vi "CalcInbetween.vi"(4 "PointY":dbl(slide) scale=-10.0..10.0, 6 "PointX":dbl(slide) scale=-10.0..10.0, 8 "Line2Y":dbl=4.0, 9 "Line2X":dbl=2.0, 10 "Line1Y":dbl format="%#_13g", 11 "Line1X":dbl format="%#_13g") -> (1 "Inbetween?":bool)   [LabVIEW 2014]
panel:
  out "Angle":dbl
  in  "cluster":T1
  out "XY Graph":cluster{dbl[], dbl[]}[](graph)
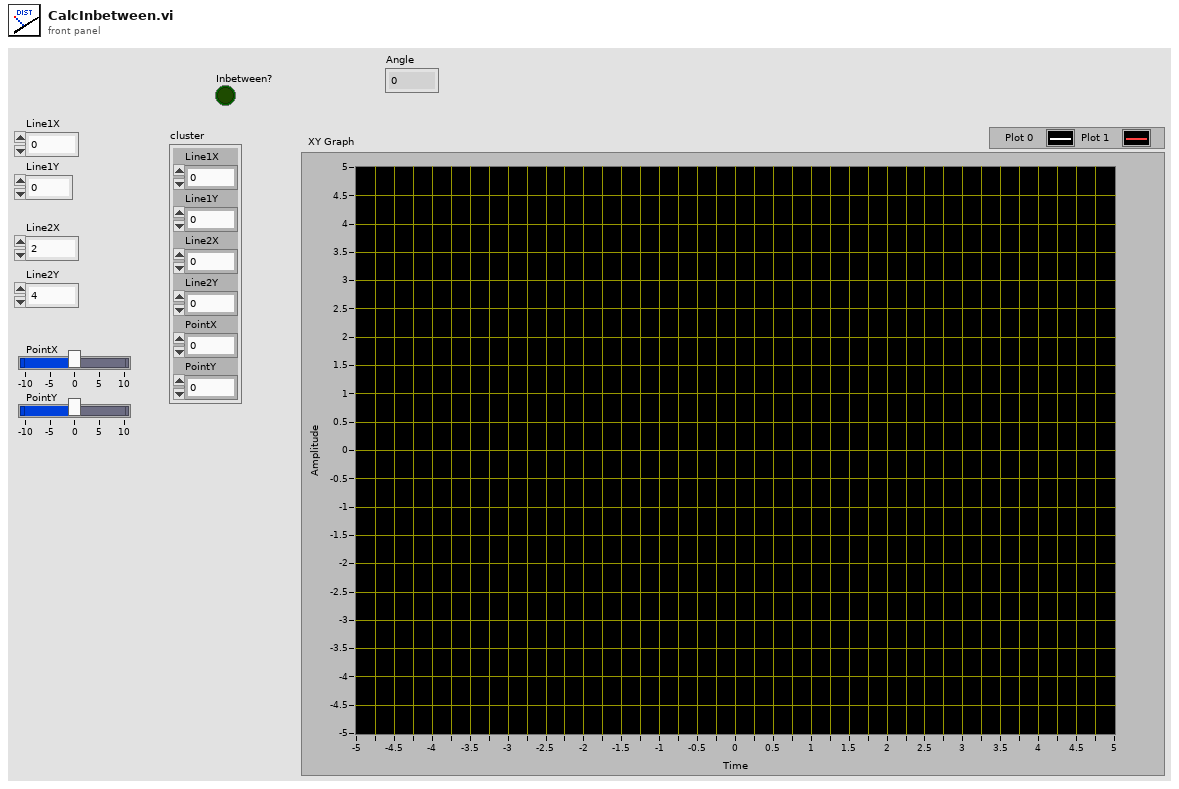
[diagram p1: front panel]
types:
  T1 = cluster{"Line1X":dbl, "Line1Y":dbl, "Line2X":dbl, "Line2Y":dbl, "PointX":dbl, "PointY":dbl}
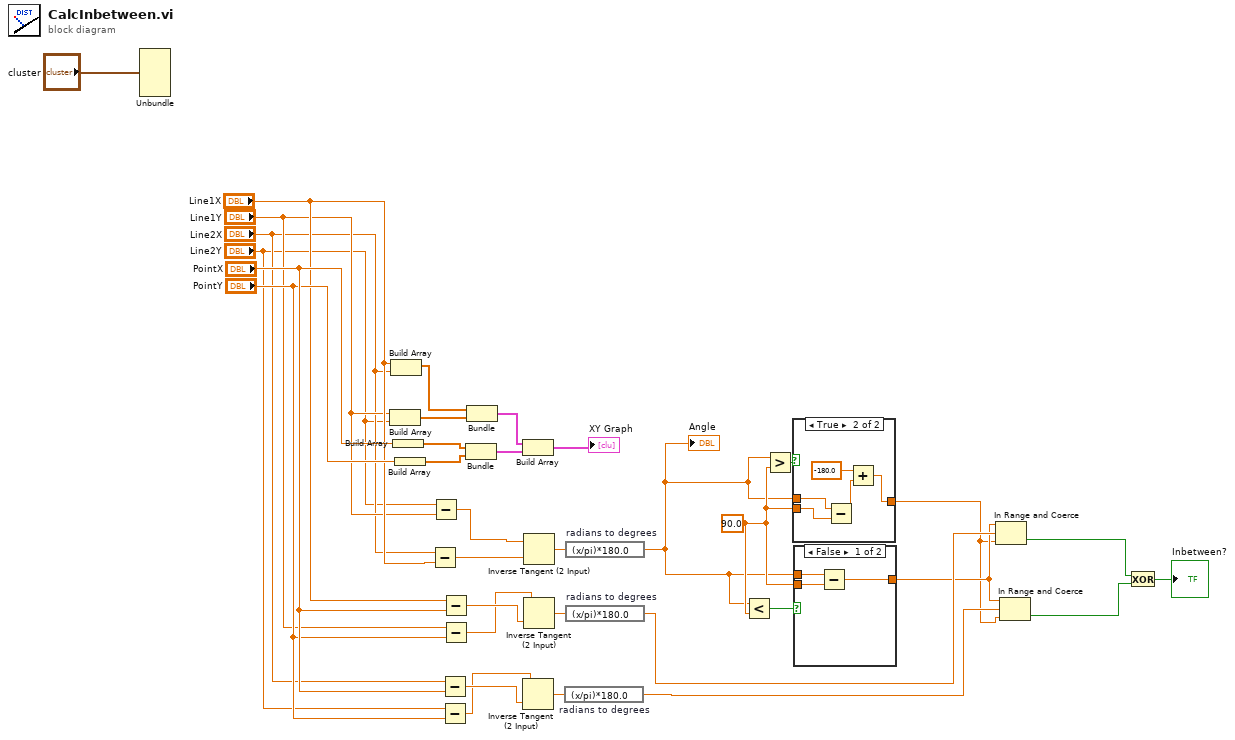
[diagram p0: block diagram]
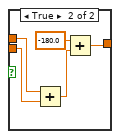
[diagram p2: hidden frame]
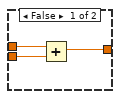
[diagram p3: hidden frame]
diagram:
  w5 = 90.0 ("y")
  n1 = Unbundle("cluster") -> ()  [unwired: 6 out]
  n2 = Build Array("Line1Y", "Line2Y") -> (w33:dbl[])
  n3 = Build Array("Line1X", "Line2X") -> (w34:dbl[])
  n4 = Build Array("PointX") -> (w32:dbl[])
  n5 = Build Array("PointY") -> (w31:dbl[])
  n6 = Subtract(x="Line2X", y="Line1X") -> (x-y=w24:dbl)
  n7 = Subtract(x="Line2Y", y="Line1Y") -> (x-y=w23:dbl)
  n8 = Subtract(x="Line2X", y="PointX") -> (x-y=w19:dbl)
  n9 = Subtract(x="Line2Y", y="PointY") -> (x-y=w18:dbl)
  n10 = Subtract(x="Line1X", y="PointX") -> (x-y=w21:dbl)
  n11 = Subtract(x="Line1Y", y="PointY") -> (x-y=w20:dbl)
  n12 = Bundle(w32, w31) -> (w30:cluster{dbl[], dbl[]})  [unwired: 1 in]
  n13 = Bundle(w34, w33) -> (w29:cluster{dbl[], dbl[]})  [unwired: 1 in]
  n14 = Build Array(w29, w30) -> (→"XY Graph":cluster{dbl[], dbl[]}[])
  n15 = Inverse Tangent (2 Input)(1:w19, 2:w18) -> (0:w22:dbl)
  n16 = Inverse Tangent (2 Input)(1:w24, 2:w23) -> (0:w26:dbl)
  n17 = Inverse Tangent (2 Input)(1:w21, 2:w20) -> (0:w25:dbl)
  n18 = expression code="(x/pi)*180.0" "radians to degrees"(w22) -> (w10:dbl)
  n19 = expression code="(x/pi)*180.0" "radians to degrees"(w26) -> (w4:dbl)
  "Angle" <- w4
  n20 = expression code="(x/pi)*180.0" "radians to degrees"(w25) -> (w11:dbl)
  n21 = Less?(x=w4, y=w5) -> (x < y?=w3:bool)
  n22 = Greater?(x=w4, y=w5) -> (0:w6:bool)
  n23 = case shown="True" w6 {
    tunnel: [w37 w40] -> w1
    tunnel: w5 -> [w36 w38]
    tunnel: w4 -> [w35 w39]
    frame False {
      n24 = Add(x=w35, y=w36) -> (x+y=w37:dbl)
    }
    frame True {
      n25 = Subtract(x=w39, y=w38) -> (x-y=w41:dbl)
      n26 = Add(x=-180.0, y=w41) -> (x+y=w40:dbl)
    }
  }
  n27 = case shown="False" w3 {
    tunnel: [w45 w49] -> w2
    tunnel: w5 -> [w44 w47]
    tunnel: w4 -> [w43 w48]
    frame False {
      n28 = Subtract(x=w43, y=w44) -> (x-y=w45:dbl)
    }
    frame True {
      n29 = Add(x=w48, y=w47) -> (x+y=w46:dbl)
      n30 = Add(x=-180.0, y=w46) -> (x+y=w49:dbl)
    }
  }
  n31 = In Range and Coerce(upper limit=w2, x=w11, lower limit=w1) -> (In Range?=w9:bool)  [unwired: 1 out]
  n32 = In Range and Coerce(upper limit=w2, x=w10, lower limit=w1) -> (In Range?=w8:bool)  [unwired: 1 out]
  n33 = Exclusive Or(1:w8, 2:w9) -> (0:→"Inbetween?":bool)
